vi "TicksToDegrees.vi"(11 "Position (ticks)":dbl) -> (3 "Position (degrees)":dbl)   [LabVIEW 2020]
panel:
  in  "Scale Factor":dbl=5.6916
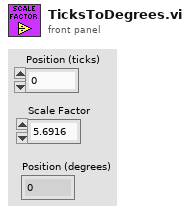
[diagram p1: front panel]
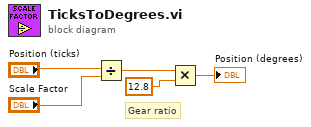
[diagram p0: block diagram]
diagram:
  # "Gear ratio"
  n1 = Divide(x="Position (ticks)", y="Scale Factor") -> (x/y=w2:dbl)
  n2 = Multiply(x=w2, y=12.8) -> (x*y=→"Position (degrees)":dbl)
